vi "CheckMeasurementsSettings.vi"(8 "error in (no error)":errorcluster, 11 "NHRDCPower in":refnum<class "NHRDCPower.lvclass">) -> (0 "error out":errorcluster, 3 "NHRDCPower out":refnum<class "NHRDCPower.lvclass">)   [LabVIEW 2018, in "AcPwrPlugins.lvlib" / "NHRDCPower.lvclass"]
doc: "This VI checks the measurement configurations to ensure that they are within the instrument specifications."
uses:
  NHRDCPower.lvclass
  C:/Projects/ICDAS - Local tetsing/NistPluggableModules/AcPwr/AcPwrPlugins/AcPwrBaseClass/AcPwrBase.lvclass
  AcPwrBaseClass/AcPwrBase.lvclass/AcPwrBase.ctl
  AcPwrBaseClass/Accessors/Read BaseMeasurements.vi
  <vilib>/Utility/error.llb/Error Cluster From Error Code.vi
  <vilib>/ErrorRing/Error Ring.xnode
panel:
  out "Time to Check Setting":u32
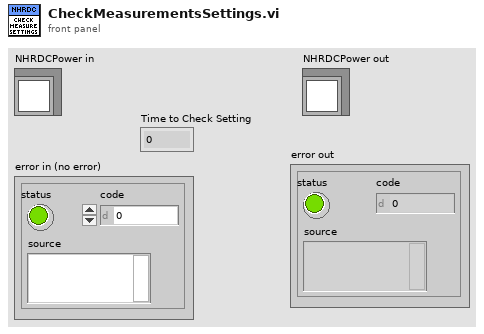
[diagram p1: front panel]
types:
  T1 = typedef "AcPwrPlugins.lvlib/AcPwrBase.lvclass/BaseMeasurements.ctl" = cluster{"Handle":string, "Name":string, "Enabled":bool, "Measurement Value":dbl, "btnMeasFetch":bool, "Chroma Hold Peak Current Measurement":bool, "Chroma Measurement Type":T2, "Chroma Protection Status String":string, "NHRDC Fetch Method":i32, "NHRDC Fetch Time (s)":sgl, "NHRDC Measurement Type":i32, "NHRGridSim Measurement Type ":enum16{"Average Current", "Max Current", "Min Current", "Average Voltage", "Max Voltage", "Min Voltage", "Average True Power", "Max True Power", "Min True Power", "Average Apparent Power", "Max Apparent Power", "Min Apparent Power", "Power Factor", "Crest Factor"}, "NHRGridSim Phase ":i32, "PPS Measurement Type ":enum16{"Voltage RMS L-N", "Voltage RMS L-L", "Frequency", "Current RMS", "Current Peak", "Crest Factor", "Power Factor", "Power VA", "Real Power"}, "PPS Channel Name":enum16{"A", "B", "C"}}[]
  T2 = typedef "AcPwrPlugins.lvlib/ChromaAcLoad.lvclass/MeasurementType.ctl" = enum16{"Voltage (Vrms or V)", "Current (Arms or A)", "Power (W)", "Peak Voltage (V)", "Peak Current (A)", "Peak Power (W)", "Frequency (Hz)", "Resistance (Ohms)", "Voltage Overshoot (V)", "Positive Peak Current (A)", "Voltage Undershoot (V)", "Negative Peak Current (A)", "Apparent Power (VA)", "Reacitive Power (VAR)", "Voltage THD", "Power Factor", "Current's Crest Factor"}
  T3 = typedef "AcPwrPlugins.lvlib/NHRDCPower.lvclass/Modules.ctl" = cluster{"Handle":string, "Name":string, "id query (Yes)":bool, "reset device (Yes)":bool, "Connected":bool, "Initial Battery Detect Voltage (0)":dbl, "SafetySettings":cluster{"SetWatchDog?":bool, "Voltage (V)":dbl, "Current (A)":dbl, "Power (W)":dbl, "Voltage Delay (s)":dbl, "Current Delay (s)":dbl, "Power Delay (s)":dbl}, "Options String":string, "Aperture Time (s)":dbl, "operating state (Off)":i32, "OutputSettings":cluster{"Voltage (V)":dbl, "Current (A)":dbl, "Resistance (Ohms)":dbl, "Power (W)":dbl, "Enable Voltage":bool, "Enable Current":bool, "Enable Resistance":bool, "Enable Power":bool, "Macro After Step Delay  (s)":dbl, "Wait Value (V, A, W)":dbl, "Enable Wait":bool, "Wait on Value":i32}, "SlewRate":cluster{"Set Voltage Rate V/S":dbl, "Set Current Rate A/S":dbl, "Set Resistance Rate R/S":dbl, "Set Power Rate W/S":dbl}, "Macro":cluster{"Save Macro?":bool, "Load Macro From File?":bool, "Run Macro Continuously?":bool, "Use Macros?":bool, "Load Macro File Path":path, "Save Macro File Path":string}, "Regulation Gain (1=100%)":dbl, "UpdatingOntheFly":bool}[]
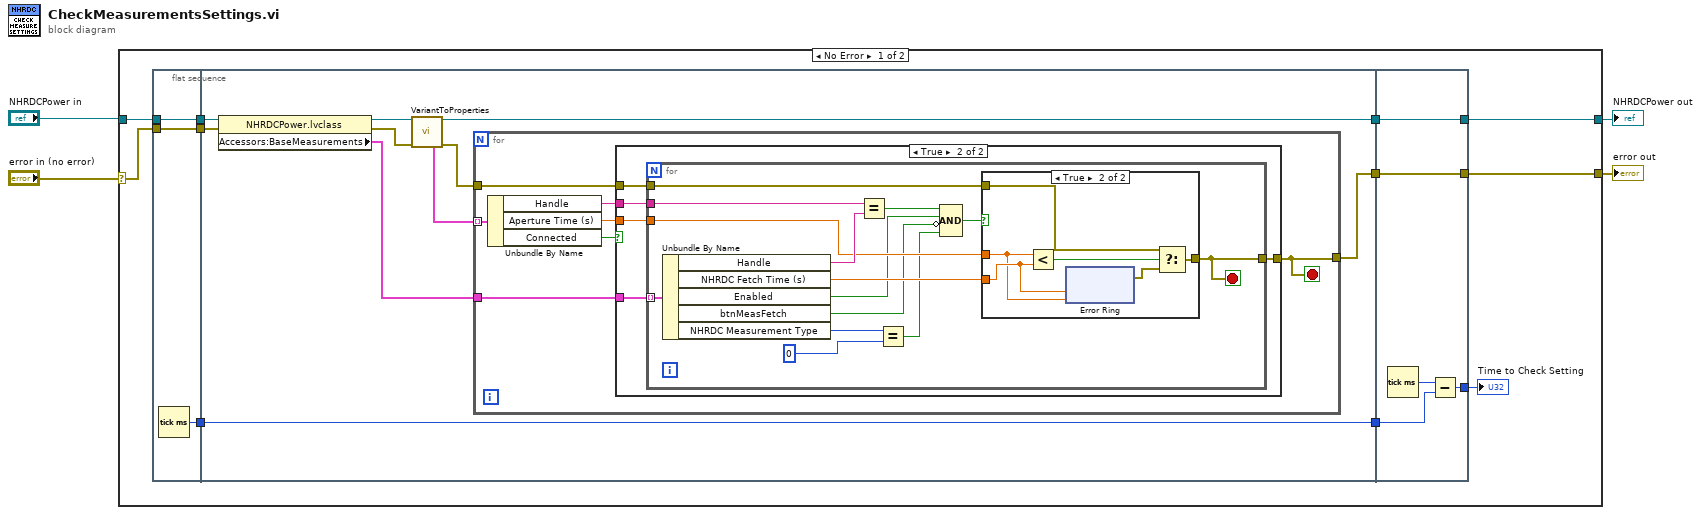
[diagram p0: block diagram]
diagram:
  n1 = case shown="No Error" "error in (no error)" {
    selector: "error in (no error)" -> [w15 w77]
    tunnel: [w13 w77] -> w1
    tunnel: [w12 w76] -> w2
    tunnel: "NHRDCPower in" -> [w14 w76]
    frame No Error {
      n2 = flat-sequence {
        tunnel: w14 -> [w17]
        tunnel: w15 -> [w18]
        tunnel: [w18] -> w9
        tunnel: [w17] -> w8
        tunnel: [w16] -> w7
        tunnel: [w25] -> w11
        tunnel: [w22] -> w10
        tunnel: w9 -> [w28]
        tunnel: w8 -> [w27]
        tunnel: w7 -> [w19]
        tunnel: [w19] -> w6
        tunnel: [w74] -> w12
        tunnel: [w75] -> w13
        tunnel: w11 -> [w75]
        tunnel: w10 -> [w74]
        tunnel: w6 -> [w72]
        tunnel: [w71] -> w5
        frame #0 {
          n3 = Tick Count (ms)() -> (millisecond timer value=w16:u32)
        }
        frame #1 {
          n4 = property class="NHRDCPower.lvclass"(reference=w27, error in=w28) -> (reference out=w23:refnum<class "NHRDCPower.lvclass">, error out=w24:errorcluster, "Accessors:BaseMeasurements"=w26:T1)
          n5 = call "VariantToProperties.vi"("NHRDCPower in"=w23, "error in (no error)"=w24) -> ("NHRDCPower out"=w22:refnum<class "NHRDCPower.lvclass">, "Modules"=w20:T3, "error out"=w21:errorcluster)  [unwired: 7 in, 4 out]
          n6 = for {
            tunnel: [w33] -> w25
            tunnel: w20 -> [w32] mode=indexing
            tunnel: w26 -> [w31]
            tunnel: w21 -> [w30]
            stop <- w33 stop-if-true
            n7 = Unbundle By Name(w32) -> ("Handle"=w35:string, "Aperture Time (s)"=w34:dbl, "Connected"=w29:bool)
            n8 = case shown="True" w29 {
              tunnel: w35 -> [_ w41]
              tunnel: w34 -> [_ w40]
              tunnel: [w36 w39] -> w33
              tunnel: w31 -> [_ w38]
              tunnel: w30 -> [w36 w37]
              frame False {
              }
              frame True {
                n9 = for {
                  tunnel: w41 -> [w55]
                  tunnel: w40 -> [w52]
                  tunnel: [w44] -> w39
                  tunnel: w38 -> [w43] mode=indexing
                  tunnel: w37 -> [w42]
                  stop <- w44 stop-if-true
                  n10 = Unbundle By Name(w43) -> ("Handle"=w54:string, "NHRDC Fetch Time (s)"=w51:sgl, "Enabled"=w49:bool, "btnMeasFetch"=w48:bool, "NHRDC Measurement Type"=w47:i32)
                  n11 = Equal?(x=w55, y=w54) -> (x = y?=w53:bool)
                  n12 = Equal?(x=w47, y=0) -> (x = y?=w45:bool)
                  n13 = Compound Arithmetic op=AND(w53, w49, invert w48, w45) -> (w50:bool)
                  n14 = case shown="True" w50 {
                    tunnel: w52 -> [_ w57]
                    tunnel: w51 -> [_ w58]
                    tunnel: [w56 w60] -> w44
                    tunnel: w42 -> [w56 w59]
                    frame False {
                    }
                    frame True {
                      n15 = Less?(x=w57, y=w58) -> (x < y?=w62:bool)
                      n16 = xnode "Error Ring"("parameter 0"=w58, "parameter 1"=w57) -> ("error out"=w61:errorcluster)
                      n17 = Select(t=w59, s=w62, f=w61) -> (s? t:f=w60:errorcluster)
                    }
                  }
                }
              }
            }
          }
        }
        frame #2 {
          n18 = Tick Count (ms)() -> (millisecond timer value=w73:u32)
          n19 = Subtract(x=w73, y=w72) -> (x-y=w71:u32)
        }
      }
      "Time to Check Setting" <- w5
    }
    frame Error {
    }
  }
  "error out" <- w1
  "NHRDCPower out" <- w2
